vi "niDTS GNSS Dut Rx Configure.vi"(0 "Dut Handle in":T2, 5 "niDTS GNSS DUT Parameters":T1={"GNSS Standard"=enum."GPS", "Frequency (Hz)"=0.0, "Power (dBm)"=0.0, "External Attenuation (dB)"=0.0, "Measurement Interval (s)"=1.0, "Enable Averaging"=FALSE, "Type Of Averaging"=enum."MEAN", "Number of Averages"=1, "Enable Traces?"=FALSE} {"External Attenuation (dB)" format="%.1g"; "Power (dBm)" format="%.1g"}, 11 "error in (no error)":errorcluster) -> (4 "Dut Handle out":T2, 15 "error out":errorcluster)   [LabVIEW 2015, in "niDTS GNSS.lvlib"]
doc: "Set the basic parameters for the WLAN TX Test. \n\nInputs:\n* Apply Additional Defaults. This allows more advanced parameters, which are dependant on the inputs, to have their default values set.\n\nCallbacks:\n* WLAN DUT Additional Defaults\n\nNote: This behavior is expected to be depricated when full parameter sets are passed as inputs and the input dependant defaults are calculated on the top parameter setting level."
uses:
  niDTS GNSS.lvlib
  Framework/Dut/Includes/niDTS Dut INC Handle.ctl
  Framework/Dut/Objects/BASE_class/niDTS Dut.lvclass
  Includes/niDTS GNSS Dut INC Parameters.ctl
  Includes/niDTS GNSS Dut INC Handle.ctl
  Objects/BASE_class/niDTS GNSS Dut.lvclass
  Framework/Logger/Objects/BASE_class/niDTS Logger.lvclass
  Framework/niDTS Framework.lvlib
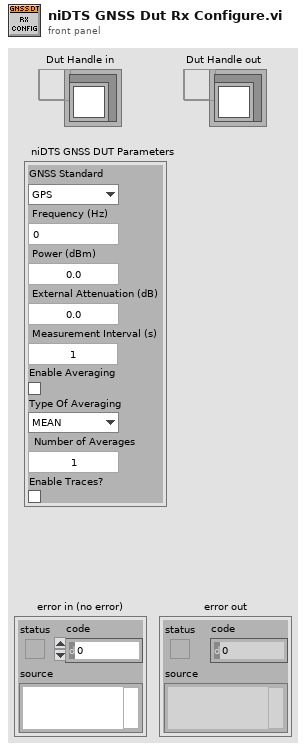
[diagram p1: front panel]
types:
  T1 = typedef "niDTS GNSS.lvlib/niDTS GNSS Dut INC Parameters.ctl" = cluster{"GNSS Standard":enum16{"GPS", "GLONASS", "Galileo", "Beidou"}, "Frequency (Hz)":dbl, "Power (dBm)":dbl, "External Attenuation (dB)":dbl, "Measurement Interval (s)":dbl, "Enable Averaging":bool, "Type Of Averaging":enum16{"MEAN", "MAX", "MIN", "MAXMIN"}, "Number of Averages":i32, "Enable Traces?":bool}
  T2 = typedef "niDTS Framework.lvlib/niDTS Dut INC Handle.ctl" = refnum<data-value>
  T3 = typedef "niDTS GNSS.lvlib/niDTS GNSS Dut INC Handle.ctl" = refnum<data-value>
  T4 = typedef "niDTS Framework.lvlib/niDTS Logger INC Handle.ctl" = refnum<data-value>
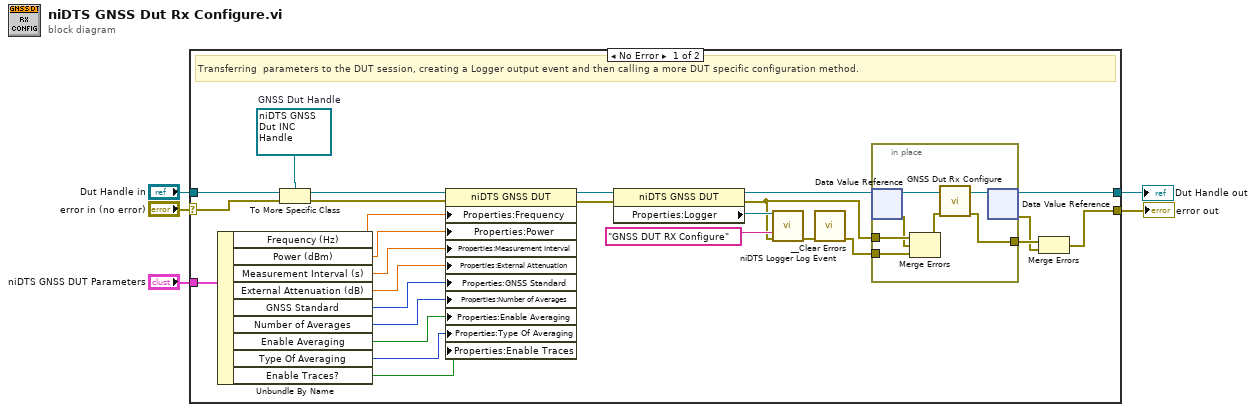
[diagram p0: block diagram]
diagram:
  n1 = case shown="No Error" "error in (no error)" {
    selector: "error in (no error)" -> [w28 w40]
    tunnel: "Dut Handle in" -> [w32 w41]
    tunnel: "niDTS GNSS DUT Parameters" -> [w29 _]
    tunnel: [w27 w41] -> w3
    tunnel: [w26 w40] -> w2
    frame No Error {
      w17 = T3 refnum  # GNSS Dut Handle
      # "Transferring  parameters to the DUT session, creating a Logger output event and then calling a more DUT specific configuration method."
      n2 = Unbundle By Name(w29) -> ("Frequency (Hz)"=w22:dbl, "Power (dBm)"=w21:dbl, "Measurement Interval (s)"=w20:dbl, "External Attenuation (dB)"=w16:dbl, "GNSS Standard"=w15:enum16{"GPS", "GLONASS", "Galileo", "Beidou"}, "Number of Averages"=w14:i32, "Enable Averaging"=w13:bool, "Type Of Averaging"=w12:enum16{"MEAN", "MAX", "MIN", "MAXMIN"}, "Enable Traces?"=w11:bool)
      n3 = To More Specific Class(target class=w17, reference=w32, error in=w28) -> (specific class reference=w31:T3, error out=w30:errorcluster)
      n4 = property class="niDTS GNSS DUT"(reference=w31, error in=w30, "Properties:Frequency"=w22, "Properties:Power"=w21, "Properties:Measurement Interval"=w20, "Properties:External Attenuation"=w16, "Properties:GNSS Standard"=w15, "Properties:Number of Averages"=w14, "Properties:Enable Averaging"=w13, "Properties:Type Of Averaging"=w12, "Properties:Enable Traces"=w11) -> (reference out=w19:T3, error out=w18:errorcluster)
      n5 = property class="niDTS GNSS DUT"(reference=w19, error in=w18) -> (reference out=w23:T3, error out=w10:errorcluster, "Properties:Logger"=w25:T4)
      n6 = call "niDTS Logger Log Event.vi"("Logger Handle"=w25, "Source/Location"="GNSS DUT RX Configure", "error in (no error)"=w10) -> ("error out"=w9:errorcluster)  [unwired: 10 in, 2 out]
      n7 = call "__Clear Errors.vi"("error in (no error)"=w9) -> ("error out"=w8:errorcluster)  [unwired: 5 in, 1 out]
      n8 = in-place {
        in-place-border: w10 -> [w35]
        in-place-border: [w36] -> w7
        in-place-border: w8 -> [w34]
        n9 = in-place-dvr #1(w23) -> (w39:refnum<class "niDTS GNSS Dut.lvclass">, w33:errorcluster)
        n10 = Merge Errors(w35, w33, w34) -> (w38:errorcluster)
        n11 = call-dynamic "GNSS Dut Rx Configure.vi"("niDTS GNSS DUT in"=w39, "error in (no error)"=w38) -> ("niDTS GNSS DUT out"=w37:refnum<class "niDTS GNSS Dut.lvclass">, "error out"=w36:errorcluster)  [unwired: 12 in]
        n12 = in-place-dvr #1(w37) -> (w27:T3, w6:errorcluster)
      }
      n13 = Merge Errors(w7, w6) -> (w26:errorcluster)
    }
    frame Error {
    }
  }
  "error out" <- w2
  "Dut Handle out" <- w3
